vi "Configure Digital All Channel.vi"(9 "Cyclic":bool, 10 "Output":bool, 11 "ADALM2000 In":u64 caption="Instrument Handle Out") -> (3 "ADALM2000 Out":u64 caption="Instrument Handle Out")   [LabVIEW 2022 SP3]
uses:
  libm2k_lv.dll
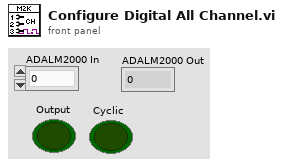
[diagram p1: front panel]
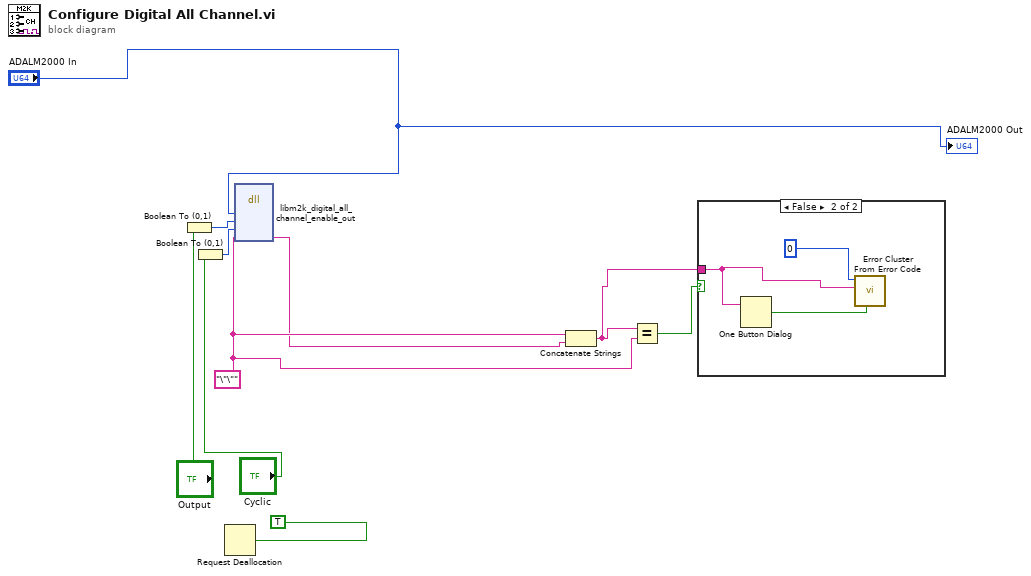
[diagram p0: block diagram]
diagram:
  w7 = "\"\""
  n1 = Boolean To (0,1)(Boolean="Output") -> (0, 1=w9:i16)
  n2 = Boolean To (0,1)(Boolean="Cyclic") -> (0, 1=w3:i16)
  n3 = Request Deallocation(TRUE ("flag")) -> ()
  n4 = dll-call lib="libm2k_lv.*" fn="libm2k_digital_all_channel_enable_out"("instance"="ADALM2000 In", "output"=w9, "cyclic"=w3, "err"=w7) -> ("err"=w4:string)  [unwired: 7 in, 2 out]
  n5 = Concatenate Strings(w7, w4) -> (w5:string)
  n6 = Equal?(x=w5, y=w7) -> (x = y?=w6:bool)
  n7 = case shown="False" w6 {
    tunnel: w5 -> [_ w11]
    frame True {
    }
    frame False {
      n8 = One Button Dialog(message=w11) -> (true=w13:bool)  [unwired: 1 in]
      n9 = call <vilib>:"Error Cluster From Error Code.vi"("show call chain? (False)"=w13, "error message (\"\")"=w11, "error code (0)"=0) -> ()  [unwired: 6 in, 1 out]
    }
  }
  "ADALM2000 Out" <- "ADALM2000 In"
